vi "GetBarStartPosition.vi"(8 "error in (no error)":errorcluster, 11 "Code128 in":refnum<class "Code128.lvclass">) -> (0 "error out":errorcluster, 2 "Start Position":cluster{"x":i16, "y":i16}={"x"=10, "y"=3}, 3 "Code128 out":refnum<class "Code128.lvclass">)   [LabVIEW 2013, in "BarCodes.lvlib" / "Code128.lvclass"]
doc: "Specifies the top-left corner of the barcode in a given image. This effectively sets the quiet space in either direction around the bar code."
uses:
  Code128.lvclass
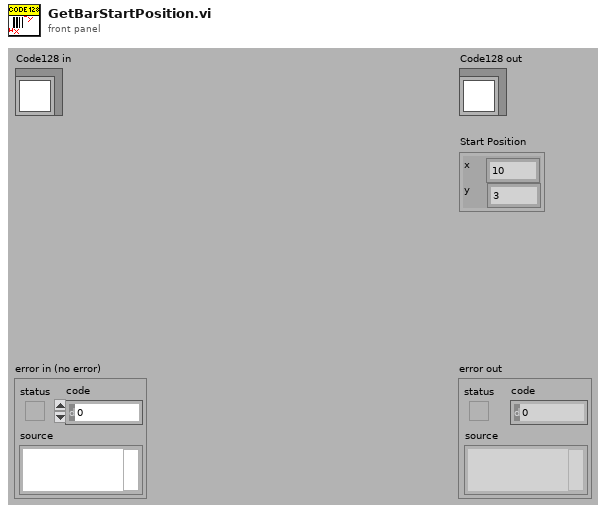
[diagram p1: front panel]
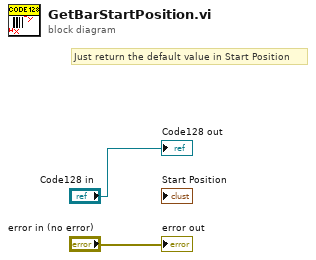
[diagram p0: block diagram]
diagram:
  # "Just return the default value in Start Position"
  "error out" <- "error in (no error)"
  "Code128 out" <- "Code128 in"
